vi "Setup UI.vi"(8 "error in (no error)":errorcluster, 10 "Set UI to input? (F)":bool, 11 "Wavelength Digikröm in":refnum<class "Wavelength Digikröm.lvclass">) -> (0 "error out":errorcluster, 3 "Wavelength Digikröm out":refnum<class "Wavelength Digikröm.lvclass">)   [LabVIEW 2017, in "Wavelength Digikröm.lvclass"]
doc: "Scanner::Setup is a constructor that has no parameters and faces the user. The Factory calls this VI to let the user configure this Scanner. It is dynamically dispatched in order to let the user choose the type as well as the options of the scanner."
panel:
  in  "Set Slits":bool
  in  "Exit Slit":dbl[unit]=9.999999999999999e-06
  in  "Entrance Slit":dbl[unit]=9.999999999999999e-06
  out "Ready":bool
  in  "Go to first point":bool
  out "Suggested Step Size":dbl
  in  "Filter":u8(ring)=1 items=["No Filter"=1, "Filter 1"=2, "Filter 2"=3, "Filter 3"=4, "Filter 4"=5, "Filter 5"=6]
  # "Digikrom DK240 Setup"
  # "Do not attempt to change\nany settings or start scan \nwhile light is off"
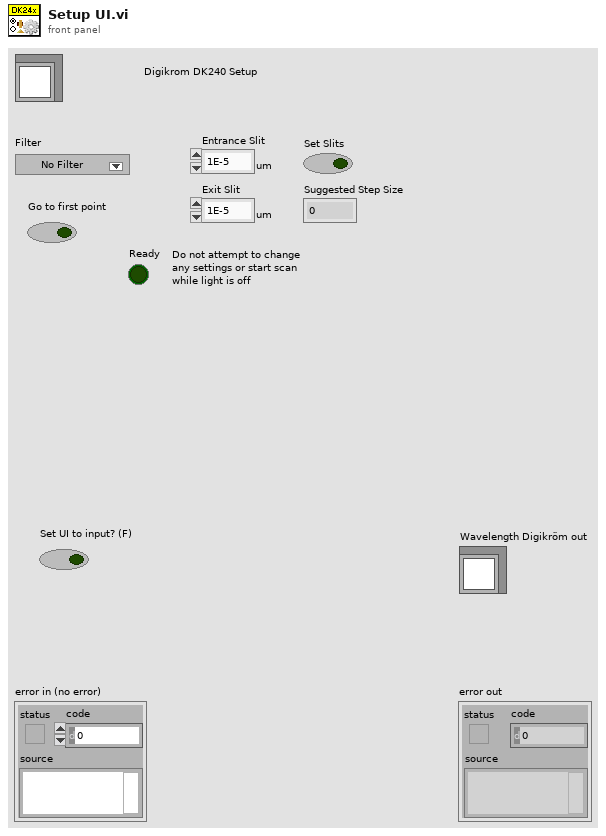
[diagram p1: front panel]
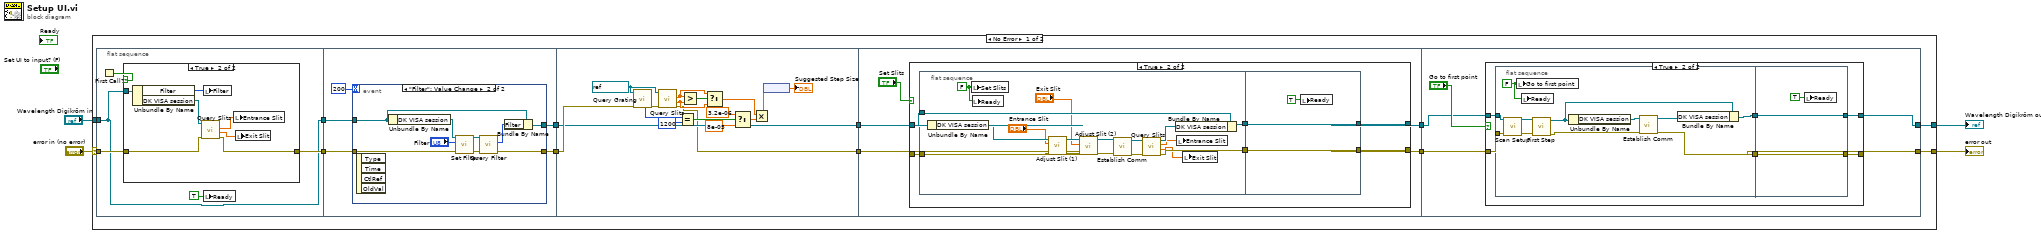
[diagram p0: block diagram]
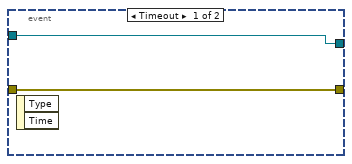
[diagram p3: hidden frame]
diagram:
  n1 = case shown="No Error" "error in (no error)" {
    selector: "error in (no error)" -> [w14 w123]
    tunnel: "Wavelength Digikröm in" -> [w16 w124]
    tunnel: [w13 w123] -> w2
    tunnel: [w12 w124] -> w1
    frame No Error {
      n2 = flat-sequence {
        tunnel: w16 -> [w17]
        tunnel: [w18] -> w15
        tunnel: w14 -> [w19]
        tunnel: [w17] -> w5
        tunnel: w15 -> [w33]
        tunnel: [w31] -> w11
        tunnel: [w30] -> w10
        tunnel: w5 -> [w32]
        tunnel: [w46] -> w9
        tunnel: [w47] -> w7
        tunnel: w10 -> [w47]
        tunnel: w11 -> [w62]
        tunnel: w9 -> [w67]
        tunnel: [w66] -> w8
        tunnel: w7 -> [w64]
        tunnel: [w65] -> w6
        tunnel: [w96] -> w12
        tunnel: [w97] -> w13
        tunnel: w8 -> [w98]
        tunnel: w6 -> [w99]
        frame #0 {
          n3 = First Call?() -> (First Call?: T/F=w20:bool)
          n4 = case shown="True" w20 {
            tunnel: w17 -> [_ w29]
            tunnel: w19 -> [w22 w26]
            tunnel: [w22 w25] -> w18
            frame False {
            }
            frame True {
              n5 = Unbundle By Name(w29) -> ("Filter"=w28:u8, "DK VISA session"=w27:refnum<visa-resource-name>)
              n6 = call "Query Slits.vi"("error in (no error)"=w26, "VISA resource name"=w27) -> ("error out"=w25:errorcluster, "CURRENT S2 WIDTH"=w23:dbl[unit], "CURRENT S1 WIDTH"=w24:dbl[unit])  [unwired: 7 out]
              n7 = local write "Filter"(w28) -> ()
              n8 = local write "Entrance Slit"(w24) -> ()
              n9 = local write "Exit Slit"(w23) -> ()
            }
          }
          n10 = local write "Ready"(TRUE ("Ready")) -> ()
        }
        frame #1 {
          n11 = event shown="[1] \"Filter\": Value Change" {
            selector: _ -> [_ _]
            dyn-events: _ -> [_ _]
            timeout: 200 -> [_ _]
            tunnel: w33 -> [w35 w44]
            tunnel: w32 -> [w36 w39]
            tunnel: [w35 w40] -> w31
            tunnel: [w36 w38] -> w30
            event Timeout {
              n12 = event-data() -> ()  [unwired: 1 in, 2 out]
            }
            event "Filter": Value Change {
              n13 = event-data() -> ()  [unwired: 1 in, 4 out]
              n14 = Unbundle By Name(w39) -> ("DK VISA session"=w43:refnum<visa-resource-name>)
              n15 = call "Set Filter.vi"("error in (no error)"=w44, "NEW FILTER"="Filter", "VISA resource name"=w43) -> ("error out"=w41:errorcluster, "VISA resource name out"=w42:refnum<visa-resource-name>)  [unwired: 7 in]
              n16 = call "Query Filter.vi"("error in (no error)"=w41, "VISA resource name"=w42) -> ("error out"=w40:errorcluster, "CURRENT FILTER"=w37:u8)  [unwired: 7 in, 1 out]
              n17 = Bundle By Name(cluster=w39, "Filter"=w37) -> (w38:refnum<class "Wavelength Digikröm.lvclass">)
            }
          }
        }
        frame #2 {
          w61 = refnum<visa-resource-name> "COM1" ("VISA resource name")
          n18 = call "Query Grating.vi"("error in (no error)"=w62, "VISA resource name"=w61) -> ("error out"=w60:errorcluster, "GR/MM"=w56:u16)  [unwired: 4 in, 4 out]
          n19 = call "Query Slits.vi"("error in (no error)"=w60, "VISA resource name"=w61) -> ("error out"=w46:errorcluster, "CURRENT S2 WIDTH"=w57:dbl[unit], "CURRENT S1 WIDTH"=w58:dbl[unit])  [unwired: 5 in, 2 out]
          n20 = Equal?(x=w56, y=u16 1200) -> (x = y?=w54:bool)
          n21 = Greater?(x=w58, y=w57) -> (0:w59:bool)
          n22 = Select(t=w58, s=w59, f=w57) -> (s? t:f=w51:dbl[unit])
          n23 = Select(t=3.2e-06, s=w54, f=8e-05) -> (s? t:f=w50:dbl)
          n24 = Multiply(x=w51, y=w50) -> (x*y=w49:dbl[unit])
          n25 = node(w49) -> (→"Suggested Step Size":dbl)
        }
        frame #3 {
          n26 = case shown="True" "Set Slits" {
            tunnel: w67 -> [w69 w75]
            tunnel: [w69 w74] -> w66
            tunnel: [w68 w73] -> w65
            tunnel: w64 -> [w68 w72]
            frame False {
            }
            frame True {
              n27 = flat-sequence {
                tunnel: w75 -> [w86]
                tunnel: w72 -> [w82]
                tunnel: [w85] -> w71
                tunnel: [w83] -> w70
                tunnel: [w94] -> w73
                tunnel: [w95] -> w74
                tunnel: w71 -> [w95]
                tunnel: w70 -> [w94]
                frame #0 {
                  w76 = FALSE ("Set Slits")
                  n28 = Unbundle By Name(w82) -> ("DK VISA session"=w84:refnum<visa-resource-name>)
                  n29 = local write "Set Slits"(w76) -> ()
                  n30 = local write "Ready"(w76) -> ()
                  n31 = call "Adjust Slit (1).vi"("error in (no error)"=w86, "SLIT WIDTH"="Entrance Slit", "VISA resource name"=w84) -> ("error out"=w89:errorcluster, "VISA resource name out"=w92:refnum<visa-resource-name>)  [unwired: 7 out]
                  n32 = call "Adjust Slit (2).vi"("error in (no error)"=w89, "SLIT WIDTH"="Exit Slit", "VISA resource name"=w92) -> ("error out"=w88:errorcluster, "VISA resource name out"=w91:refnum<visa-resource-name>)  [unwired: 7 out]
                  n33 = call "Establish Comm.vi"("error in (no error)"=w88, "VISA resource name"=w91) -> ("error out"=w87:errorcluster, "VISA resource name out"=w90:refnum<visa-resource-name>)  [unwired: 8 in]
                  n34 = call "Query Slits.vi"("error in (no error)"=w87, "VISA resource name"=w90) -> ("error out"=w85:errorcluster, "CURRENT S2 WIDTH"=w79:dbl[unit], "CURRENT S1 WIDTH"=w80:dbl[unit], "VISA resource name out"=w81:refnum<visa-resource-name>)  [unwired: 6 out]
                  n35 = Bundle By Name(cluster=w82, "DK VISA session"=w81) -> (w83:refnum<class "Wavelength Digikröm.lvclass">)
                  n36 = local write "Entrance Slit"(w80) -> ()
                  n37 = local write "Exit Slit"(w79) -> ()
                }
                frame #1 {
                  n38 = local write "Ready"(TRUE ("Ready")) -> ()
                }
              }
            }
          }
        }
        frame #4 {
          n39 = case shown="True" "Go to first point" {
            tunnel: w99 -> [w102 w107]
            tunnel: [w102 w105] -> w96
            tunnel: [w101 w106] -> w97
            tunnel: w98 -> [w101 w108]
            frame False {
            }
            frame True {
              n40 = flat-sequence {
                tunnel: w108 -> [w119]
                tunnel: w107 -> [w118]
                tunnel: [w112] -> w104
                tunnel: [w110] -> w103
                tunnel: [w121] -> w105
                tunnel: [w122] -> w106
                tunnel: w104 -> [w122]
                tunnel: w103 -> [w121]
                frame #0 {
                  w115 = FALSE ("Go to first point")
                  n41 = call-dynamic "Scan Setup.vi"("error in (no error)"=w119, "Wavelength Digikröm in"=w118) -> ("error out"=w117:errorcluster, "Wavelength Digikröm out"=w116:refnum<class "Wavelength Digikröm.lvclass">)  [unwired: 8 in]
                  n42 = local write "Go to first point"(w115) -> ()
                  n43 = local write "Ready"(w115) -> ()
                  n44 = call-dynamic "First Step.vi"("error in (no error)"=w117, "Wavelength Digikröm.lvclass in"=w116) -> ("error out"=w113:errorcluster, "Wavelength Digikröm.lvclass out"=w111:refnum<class "Wavelength Digikröm.lvclass">)  [unwired: 7 in, 1 out]
                  n45 = Unbundle By Name(w111) -> ("DK VISA session"=w114:refnum<visa-resource-name>)
                  n46 = call "Establish Comm.vi"("error in (no error)"=w113, "VISA resource name"=w114) -> ("error out"=w112:errorcluster, "VISA resource name out"=w109:refnum<visa-resource-name>)  [unwired: 8 in]
                  n47 = Bundle By Name(cluster=w111, "DK VISA session"=w109) -> (w110:refnum<class "Wavelength Digikröm.lvclass">)
                }
                frame #1 {
                  n48 = local write "Ready"(TRUE ("Ready")) -> ()
                }
              }
            }
          }
        }
      }
    }
    frame Error {
    }
  }
  "error out" <- w2
  "Wavelength Digikröm out" <- w1
